vi "send_Brain.vi"   [LabVIEW 2013]
uses:
  <vilib>/NXT/Block Support/NXT_MessageMailbox.ctl
  <vilib>/NXT/Dual Mode Library/BT/BlueTooth_Write_Num.vi
  <vilib>/NXT/Dual Mode Library/Sound/Tone.vi
  <vilib>/NXT/Dual Mode Library/Display/drawNumber.vi
types:
  T1 = typedef "NXT_MessageMailbox.ctl" = u8
  T2 = typedef "LVHSConnector.ctl" = refnum<class "BrickReference.lvclass">
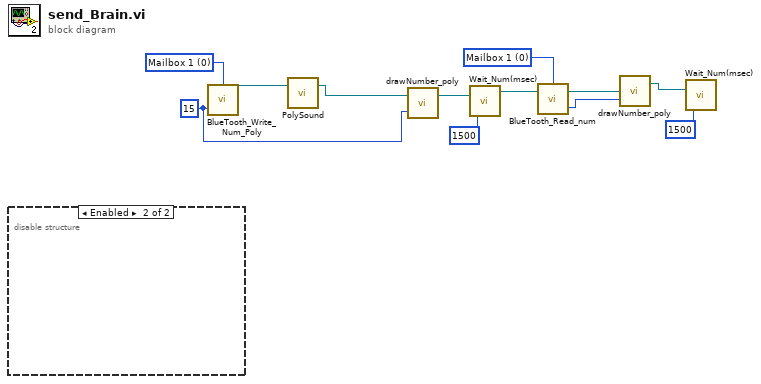
[diagram p0: block diagram]
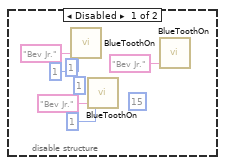
[diagram p2: hidden frame]
diagram:
  w2 = T1 0 items=["Mailbox 1", "Mailbox 2", "Mailbox 3", "Mailbox 4", "Mailbox 5", "Mailbox 6", "Mailbox 7", "Mailbox 8", "Mailbox 9", "Mailbox 10"] ("Mailbox")
  w5 = 15 ("Message")
  w12 = T1 0 items=["Mailbox 1", "Mailbox 2", "Mailbox 3", "Mailbox 4", "Mailbox 5", "Mailbox 6", "Mailbox 7", "Mailbox 8", "Mailbox 9", "Mailbox 10"] ("Mailbox")
  n1 = disable-structure shown="Enabled" {
    frame Disabled {
      (unwired) u8 1 ("Connection")
      (unwired) u8 1 ("Connection")
      (unwired) 15 ("Message")
      n2 = call "BlueToothOn.vi"("Connection"=u8 1, "Partner Name"="Bev Jr.") -> ("NXT/EV3 2"=w16:T2)  [unwired: 1 in, 3 out]
      n3 = call "BlueToothOn.vi"("Connection"=u8 1, "Partner Name"="Bev Jr.") -> ("NXT/EV3 2"=w19:T2)  [unwired: 1 in, 3 out]
      n4 = call "BlueToothOn.vi"("Partner Name"="Bev Jr.") -> ("NXT/EV3 2"=w14:T2)  [unwired: 2 in, 3 out]
    }
    frame Enabled {
    }
  }
  n5 = call-poly <vilib>:"BlueTooth_Write_Num_Poly.vi"("Message"=w5, "Mailbox"=w12) -> ("NXT/EV3"=w11:T2)  [unwired: 2 in]
  n6 = call-poly <vilib>:"PolySound.vi"("NXT/EV3"=w11) -> ("NXT/EV3"=w6:T2)  [unwired: 3 in]
  n7 = call-poly <vilib>:"drawNumber_poly.vi"("number"=w5, "NXT/EV3"=w6) -> ("NXT/EV3"=w9:T2)  [unwired: 2 in]
  n8 = call <vilib>:"Wait_Num(msec).vi"("Time (100 msec)"=u32 1500, "NXT/EV3"=w9) -> ("NXT/EV3"=w8:T2)  [unwired: 2 in]
  n9 = call <vilib>:"BlueTooth_Read_num.vi"("NXT/EV3"=w8, "Mailbox"=w2) -> ("Message"=w1:i32, "NXT/EV3"=w10:T2)  [unwired: 1 in]
  n10 = call-poly <vilib>:"drawNumber_poly.vi"("number"=w1, "NXT/EV3"=w10) -> ("NXT/EV3"=w3:T2)  [unwired: 2 in]
  n11 = call <vilib>:"Wait_Num(msec).vi"("Time (100 msec)"=u32 1500, "NXT/EV3"=w3) -> ()  [unwired: 2 in, 1 out]
